vi "Command.vi"(8 "error in (no error)":errorcluster, 10 "command":string, 11 "VI Probe in":refnum<class "PL MKS VI Probe.lvclass">) -> (0 "error out":errorcluster, 2 "response data":string, 3 "VI Probe out":refnum<class "PL MKS VI Probe.lvclass">)   [LabVIEW 2015, in "PL MKS VI Probe.lvclass"]
doc: "Sends <b>command</b> to device and returns <b>response data</b>."
uses:
  PL MKS VI Probe.lvclass
  PL MKS VI Probe.lvclass/PL MKS VI Probe.ctl
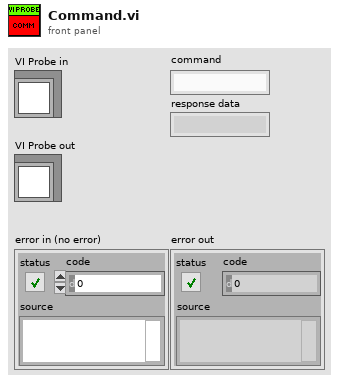
[diagram p1: front panel]
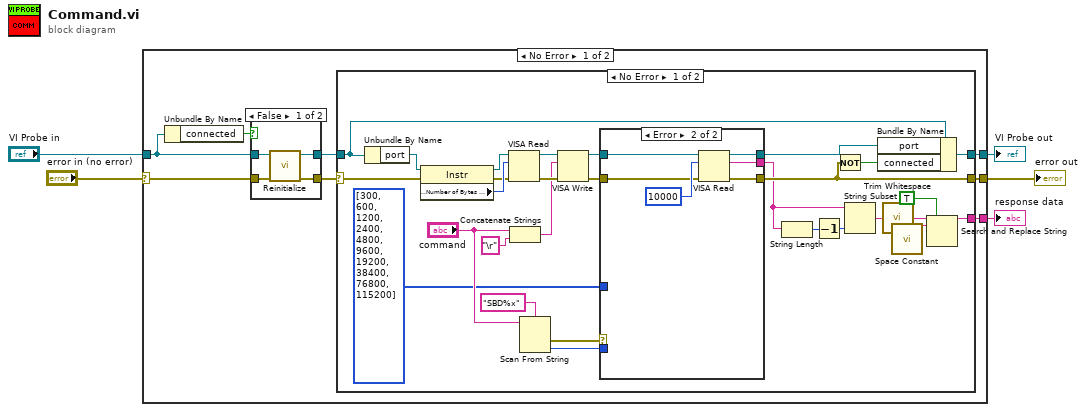
[diagram p0: block diagram]
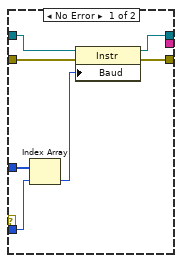
[diagram p2: hidden frame]
diagram:
  n1 = case shown="No Error" "error in (no error)" {
    selector: "error in (no error)" -> [w11 w65]
    tunnel: "VI Probe in" -> [w12 w64]
    tunnel: [w8 w65] -> w2
    tunnel: [w7 w64] -> w3
    tunnel: [w6 _] -> w1
    frame No Error {
      n2 = Unbundle By Name(w12) -> ("connected"=w13:bool)
      n3 = case shown="False" w13 {
        tunnel: w12 -> [w61 w63]
        tunnel: w11 -> [w60 w62]
        tunnel: [w59 w63] -> w9
        tunnel: [w58 w62] -> w10
        frame False {
          n4 = call "Reinitialize.vi"("error in (no error)"=w60, "VI Probe in"=w61) -> ("error out"=w58:errorcluster, "VI Probe out"=w59:refnum<class "PL MKS VI Probe.lvclass">)  [unwired: 8 in]
        }
        frame True {
        }
      }
      n5 = case shown="No Error" w10 {
        selector: w10 -> [w35 w57]
        tunnel: w9 -> [w42 w56]
        tunnel: [w15 w57] -> w8
        tunnel: [w33 w56] -> w7
        tunnel: [w17 _] -> w6
        frame No Error {
          n6 = Unbundle By Name(w42) -> ("port"=w36:refnum<visa-resource-name>)
          n7 = property class="Instr"(reference=w36, error in=w35) -> (reference out=w39:refnum<visa-resource-name>, error out=w34:errorcluster, "Serial Settings:Number of Bytes at Serial Port"=w40:u32)
          n8 = VISA Read(VISA resource name=w39, byte count=w40, error in (no error)=w34) -> (VISA resource name out=w38:refnum<visa-resource-name>, error out=w37:errorcluster)  [unwired: 2 out]
          n9 = Concatenate Strings("command", "\r" ("string")) -> (w22:string)
          n10 = Scan From String(format string="SBD%x", input string="command") -> (error out=w20:errorcluster, output 1=w19:u32)  [unwired: 3 in, 2 out]
          n11 = VISA Write(VISA resource name=w38, write buffer=w22, error in (no error)=w37) -> (VISA resource name out=w26:refnum<visa-resource-name>, error out=w25:errorcluster)  [unwired: 1 out]
          n12 = case shown="Error" w20 {
            tunnel: w26 -> [w47 w54]
            tunnel: w25 -> [w46 w51]
            tunnel: w19 -> [w48 _]
            tunnel: u32[] [300, 600, 1200, 2400, 4800, 9600, 19200, 38400, 76800, 115200] -> [w49 _]
            tunnel: [w44 w52] -> w15
            tunnel: [w43 w53] -> w16
            tunnel: [_ w50] -> w14
            frame No Error {
              n13 = Index Array(array=w49, index=w48) -> (element=w45:u32)
              n14 = property class="Instr"(reference=w47, error in=w46, "Baud"=w45) -> (reference out=w43:refnum<visa-resource-name>, error out=w44:errorcluster)
            }
            frame Error {
              n15 = VISA Read(VISA resource name=w54, byte count=u32 10000, error in (no error)=w51) -> (VISA resource name out=w53:refnum<visa-resource-name>, read buffer=w50:string, error out=w52:errorcluster)  [unwired: 1 out]
            }
          }
          n16 = String Length(string=w14) -> (length=w27:i32)
          n17 = Decrement(x=w27) -> (x-1=w28:i32)
          n18 = Not(x=w15) -> (.not. x?=w41:bool)
          n19 = String Subset(string=w14, length (rest)=w28) -> (substring=w31:string)  [unwired: 1 in]
          n20 = Bundle By Name(cluster=w42, "port"=w16, "connected"=w41) -> (w33:refnum<class "PL MKS VI Probe.lvclass">)
          n21 = call <vilib>:"Trim Whitespace.vi"("string"=w31) -> ("trimmed string"=w32:string)  [unwired: 1 in]
          n22 = call <vilib>:"Space Constant.vi"() -> ("String"=w29:string)
          n23 = Search and Replace String(replace all?=TRUE ("replace all? (F)"), input string=w32, search string=w29) -> (result string=w17:string)  [unwired: 5 in, 3 out]
        }
        frame Error {
        }
      }
    }
    frame Error {
    }
  }
  "VI Probe out" <- w3
  "error out" <- w2
  "response data" <- w1
